vi "exp seq exec logic.vi"(0 "exp exec":T2={"data file"={"autosave"=FALSE, "File refnum"=refnum, "data file path"=path ""}, "T log file"={"File refnum"=refnum, "T log file path"=path "", "exists"=FALSE}, "exp seq"={"wave params"={"Num of avg"=0, "Num points"=0, "Meas rate (Hz)"=0.0}, "Setpoints"=[], "#"=0, "index"=0, "elapsed time (s)"=0.0, "set time (s)"=0.0, "min settle (s)"=30.0, " Exec Status"=enum."Settling"}, "error"={"status"=FALSE, "code"=0, "source"=""}}, 5 "x":bool, 11 "early exit":bool) -> (4 "exit":bool, 15 "Experimental Sequence":T1)   [LabVIEW 2019]
doc: "This is a Bug C(T) subVI.\n\nIt handles the exit logic for the executive thread.\n\nPaul K Dixon\nP3600\nCSUSB Physics"
uses:
  typedefs/PID exec cluster.ctl
  typedefs/data file info.ctl
  typedefs/bug temp file info.ctl
  typedefs/exp seq cluster.ctl
  typedefs/wvfm acq params.ctl
  typedefs/bug meas status.ctl
  typedefs/exp sequence.ctl
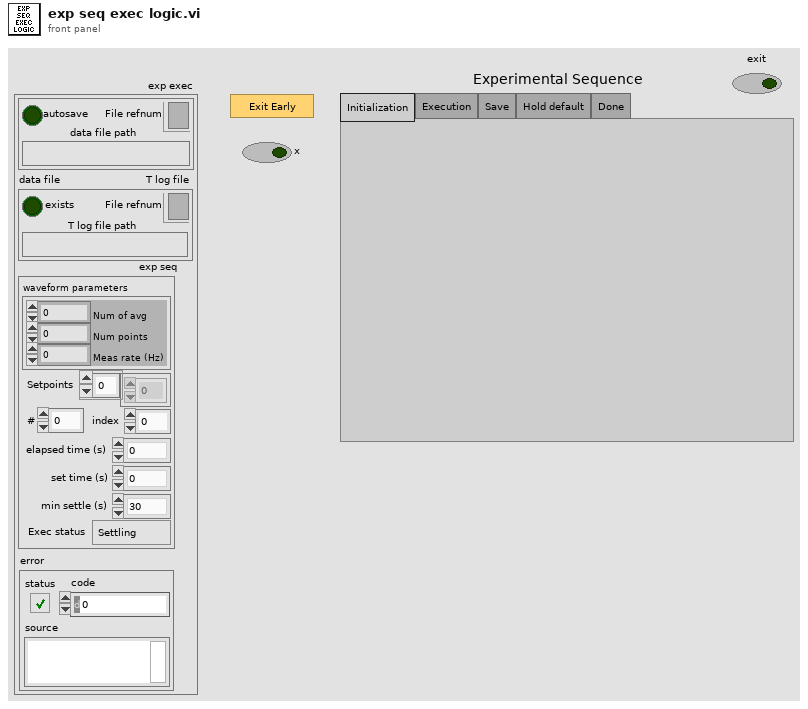
[diagram p1: front panel]
types:
  T1 = typedef "exp sequence.ctl" = enum32{"Initialization", "Execution", "Save", "Hold default", "Done"}
  T2 = typedef "PID exec cluster.ctl" = cluster{"data file":T3, "T log file":T4, "exp seq":T5, "error":errorcluster}
  T3 = typedef "data file info.ctl" = cluster{"autosave":bool, "File refnum":refnum<file>, "data file path":path}
  T4 = typedef "bug temp file info.ctl" = cluster{"File refnum":refnum<file>, "T log file path":path, "exists":bool}
  T5 = typedef "exp seq cluster.ctl" = cluster{"wave params":T6, "Setpoints":dbl[], "#":i32, "index":i32, "elapsed time (s)":dbl, "set time (s)":dbl, "min settle (s)":dbl, " Exec Status":T7}
  T6 = typedef "wvfm acq params.ctl" = cluster{"Num of avg":i32, "Num points":i32, "Meas rate (Hz)":dbl}
  T7 = typedef "bug meas status.ctl" = enum32{"Settling", "Measuring", "Holding", "Exit"}
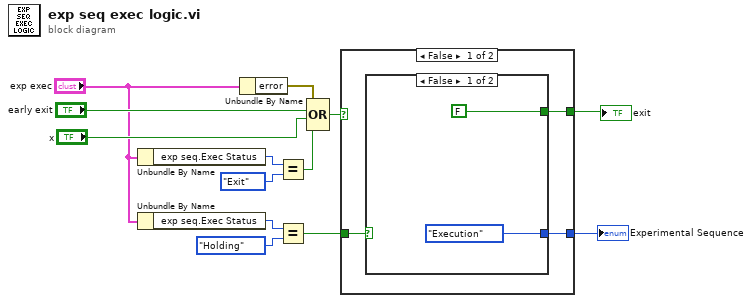
[diagram p0: block diagram]
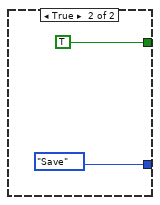
[diagram p2: hidden frame]
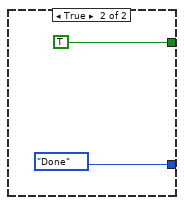
[diagram p3: hidden frame]
diagram:
  n1 = Unbundle By Name("exp exec") -> ("exp seq.Exec Status"=w3:T7)
  n2 = Unbundle By Name("exp exec") -> ("exp seq.Exec Status"=w10:T7)
  n3 = Unbundle By Name("exp exec") -> ("error"=w12:errorcluster)
  n4 = Equal?(x=w3, y=bug_meas_status."Exit" ("exp seq. Exec Status")) -> (x = y?=w1:bool)
  n5 = Equal?(x=w10, y=bug_meas_status."Holding" ("exp seq. Exec Status")) -> (x = y?=w6:bool)
  n6 = Compound Arithmetic op=OR(w12, "early exit", "x", w1) -> (w7:bool)
  n7 = case shown="False" w7 {
    tunnel: [w15 exp_sequence."Done" ("Experimental Sequence")] -> w8
    tunnel: w6 -> [w16 _]
    tunnel: [w14 TRUE ("exit")] -> w5
    frame False {
      n8 = case shown="False" w16 {
        tunnel: [exp_sequence."Execution" ("t") exp_sequence."Save" ("t")] -> w15
        tunnel: [FALSE ("exit") TRUE ("exit")] -> w14
        frame False {
        }
        frame True {
        }
      }
    }
    frame True {
    }
  }
  "exit" <- w5
  "Experimental Sequence" <- w8
